vi "Address Input Verification.vi"(3 "Error In (No Error)":errorcluster, 4 "Error if Bad? (True)":bool=TRUE, 5 "Sensor Address In (a)":string="a") -> (0 "Error Out":errorcluster, 2 "Address Valid":bool)   [LabVIEW 2016, in "SDI-12.lvlib"]
doc: "Verifies that address provided by user input is a *single* ASCII character in one of the following ranges:\n1. 0-9 (ASCII, not numeric)\n2. A-Z\n3. a-z"
uses:
  SDI-12.lvlib
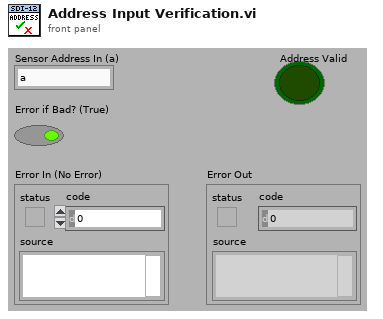
[diagram p1: front panel]
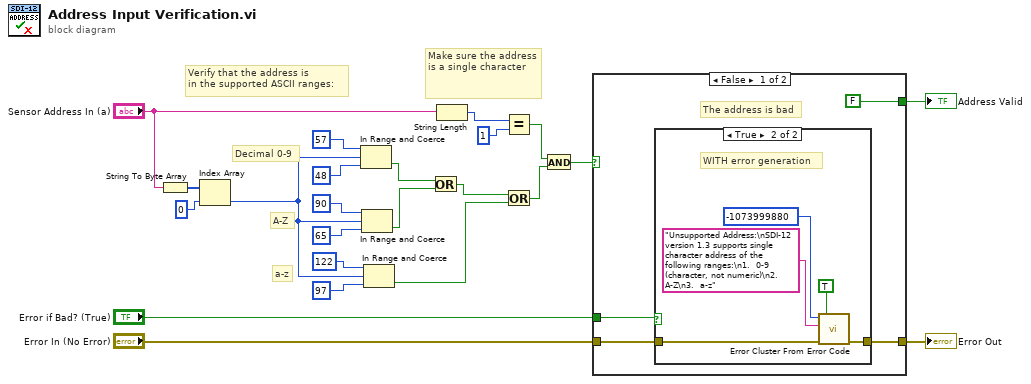
[diagram p0: block diagram]
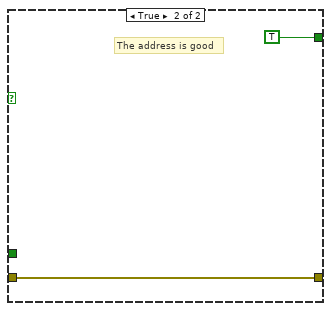
[diagram p3: hidden frame]
diagram:
  # "Verify that the address is\nin the supported ASCII ranges:"
  # "Make sure the address \nis a single character"
  # "a-z"
  # "A-Z"
  # "Decimal 0-9"
  n1 = String To Byte Array(string="Sensor Address In (a)") -> (unsigned byte array=w14:u8[])
  n2 = Index Array(array=w14, index=0) -> (element=w23:u8)
  n3 = In Range and Coerce(upper limit=u8 57, x=w23, lower limit=u8 48) -> (In Range?=w4:bool)  [unwired: 1 out]
  n4 = In Range and Coerce(upper limit=u8 90 ("lower limit"), x=w23, lower limit=u8 65) -> (In Range?=w3:bool)  [unwired: 1 out]
  n5 = In Range and Coerce(upper limit=u8 122 ("lower limit"), x=w23, lower limit=u8 97) -> (In Range?=w2:bool)  [unwired: 1 out]
  n6 = Or(x=w4, y=w3) -> (x .or. y?=w22:bool)
  n7 = String Length(string="Sensor Address In (a)") -> (length=w9:i32)
  n8 = Equal?(x=w9, y=1) -> (x = y?=w11:bool)
  n9 = Or(x=w22, y=w2) -> (x .or. y?=w12:bool)
  n10 = And(x=w11, y=w12) -> (x .and. y?=w5:bool)
  n11 = case shown="False" w5 {
    tunnel: [FALSE TRUE] -> w8
    tunnel: "Error In (No Error)" -> [w27 w35]
    tunnel: [w26 w35] -> w6
    tunnel: "Error if Bad? (True)" -> [w24 _]
    frame False {
      # "The address is bad"
      n12 = case shown="True" w24 {
        tunnel: w27 -> [w28 w29]
        tunnel: [w28 w30] -> w26
        frame False {
          # "Without error generation"
        }
        frame True {
          # "WITH error generation"
          n13 = call <vilib>:"Error Cluster From Error Code.vi"("show call chain? (False)"=TRUE, "error in (no error)"=w29, "error message (\"\")"="Unsupported Address:\nSDI-12 version 1.3 supports single character address of the following ranges:\n1.  0-9 (character, not numeric)\n2.  A-Z\n3.  a-z" ("Source (VI Name)"), "error code (0)"=-1073999880 ("Code")) -> ("error out"=w30:errorcluster)  [unwired: 5 in]
        }
      }
    }
    frame True {
      # "The address is good"
    }
  }
  "Address Valid" <- w8
  "Error Out" <- w6
